vi "Tag for JSON Text.vi"() -> (3 "Tag for JSON text":string)   [LabVIEW 2011, in "Variant JSON.lvlib"]
uses:
  Variant JSON.lvlib
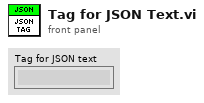
[diagram p1: front panel]
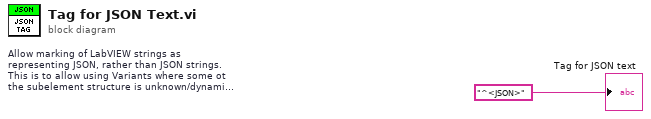
[diagram p0: block diagram]
diagram:
  w1 = "^<JSON>"  # Allow marking of LabVIEW strings as representing JSON, rather than JSON strings. This is to allow using Variants where some ot the subelement structure is unknown/dynamic -- JDP, April 2014
  "Tag for JSON text" <- w1
